vi "Actor Core.vi"(8 "error in":errorcluster, 11 "Bottom in":refnum<class "Bottom.lvclass">) -> (0 "error out":errorcluster, 3 "Actor out":refnum<class "Actor.lvclass">)   [LabVIEW 2023, in "Bottom.lvlib" / "Bottom.lvclass"]
doc: "The bottom panel actor is an abstraction that provides the actor framework panel size definitions."
uses:
  Project/Bottom.lvclass
  builds/Engine/Actor Framework.lvlibp/1abvi3w/vi.lib/ActorFramework/Actor/Actor.lvclass
  builds/Engine/Engine.lvlibp/Project/Engine.lvclass
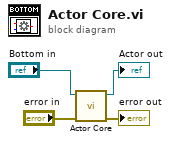
[diagram p0: block diagram]
diagram:
  n1 = call-parent "Actor Core.vi"("error in"="error in", "State Actor in"="Bottom in") -> ("error out"=→"error out":errorcluster, "Actor out"=→"Actor out":refnum<class "Actor.lvclass">)  [unwired: 8 in]
